vi "SetCalInfo.vi"(8 "CalRotateImage":T1, 9 "CalibrationTemplate":T1, 10 "Image Calibration":bool, 11 "Vision_Image":T1) -> (1 "Not an Image?":bool, 3 "ImageRef Out":T1)   [LabVIEW 2019]
uses:
  <vilib>/vision/Image Controls.llb/IMAQ Image.ctl
  <vilib>/vision/NI_Vision_Development_Module.lvlib
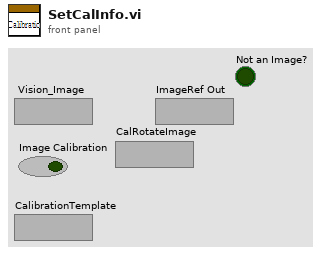
[diagram p1: front panel]
types:
  T1 = typedef "IMAQ Image.ctl" = refnum<image>
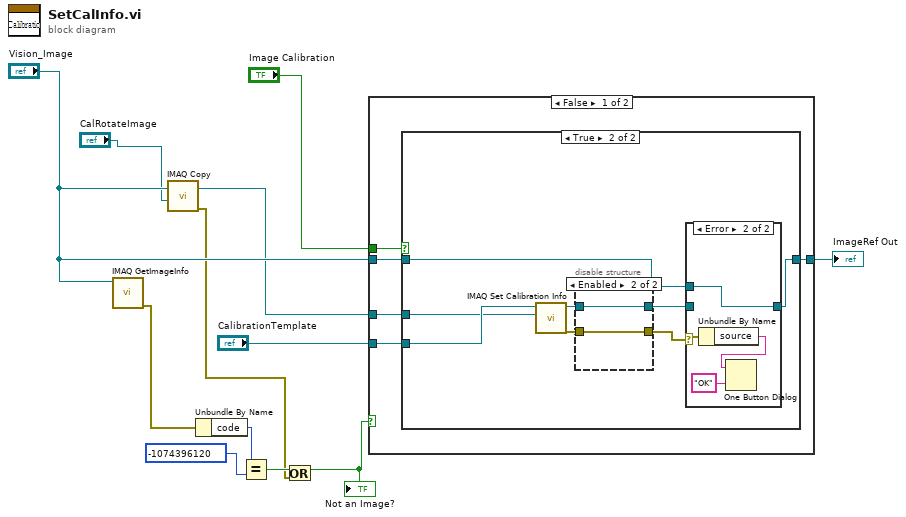
[diagram p0: block diagram]
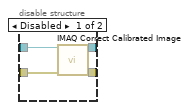
[diagram p3: hidden frame]
diagram:
  n1 = call "IMAQ GetImageInfo"("Image"="Vision_Image") -> ("error out"=w8:errorcluster)  [unwired: 3 in, 7 out]
  n2 = call "IMAQ Copy"("Image Dst"="CalRotateImage", "Image Src"="Vision_Image") -> ("error out"=w3:errorcluster, "Image Dst Out"=w2:T1)  [unwired: 4 in]
  n3 = Unbundle By Name(w8) -> ("code"=w10:i32)
  n4 = Equal?(x=w10, y=-1074396120) -> (x = y?=w7:bool)
  n5 = Or(x=w7, y=w3) -> (x .or. y?=w4:bool)
  "Not an Image?" <- w4
  n6 = case shown="False" w4 {
    tunnel: [w17 w38] -> w12
    tunnel: "CalibrationTemplate" -> [w16 _]
    tunnel: "Image Calibration" -> [w15 _]
    tunnel: "Vision_Image" -> [w14 w38]
    tunnel: w2 -> [w13 _]
    frame False {
      n7 = case shown="True" w15 {
        tunnel: [w18 w25] -> w17
        tunnel: w16 -> [_ w26]
        tunnel: w14 -> [w18 w20]
        tunnel: w13 -> [_ w19]
        frame False {
        }
        frame True {
          n8 = call "IMAQ Set Calibration Info"("Image Dst"=w19, "Image Src"=w26) -> ("error out"=w23:errorcluster, "Calibrated Image"=w24:T1)  [unwired: 2 in, 6 out]
          n9 = disable-structure shown="Enabled" {
            disable-tunnel: w24 -> [w30 w32]
            disable-tunnel: w23 -> [w29 w31]
            disable-tunnel: [w28 w31] -> w22
            disable-tunnel: [w27 w32] -> w21
            frame Disabled {
              n10 = call "IMAQ Correct Calibrated Image"("error in (no error)"=w29, "Image Src"=w30) -> ("error out"=w28:errorcluster, "Corrected Image"=w27:T1)  [unwired: 5 in, 3 out]
            }
            frame Enabled {
            }
          }
          n11 = case shown="Error" w22 {
            selector: w22 -> [_ w36]
            tunnel: w21 -> [w33 _]
            tunnel: [w33 w37] -> w25
            tunnel: w20 -> [_ w37]
            frame No Error {
            }
            frame Error {
              n12 = Unbundle By Name(w36) -> ("source"=w35:string)
              n13 = One Button Dialog(message=w35, button name ("OK")="OK") -> ()  [unwired: 1 out]
            }
          }
        }
      }
    }
    frame True {
    }
  }
  "ImageRef Out" <- w12
